vi "phase.vi"(1 "Phase":dbl) -> (0 "Phase Byte":u8=127 format="%08b")   [LabVIEW 2015]
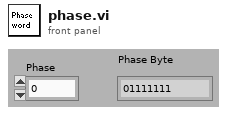
[diagram p1: front panel]
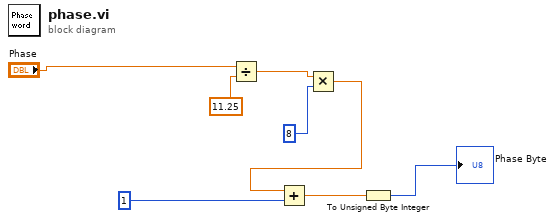
[diagram p0: block diagram]
diagram:
  n1 = Divide(x="Phase", y=11.25) -> (x/y=w6:dbl)
  n2 = Multiply(x=w6, y=8) -> (x*y=w4:dbl)
  n3 = Add(x=w4, y=1) -> (x+y=w3:dbl)
  n4 = To Unsigned Byte Integer(number=w3) -> (unsigned 8bit integer=→"Phase Byte":u8)
